vi "Apply Light-Dark Controls Visibility.vi"(8 "Error In":errorcluster, 9 "Dark Controls":refnum<vi>[](array[refnum]), 10 "Light Controls":refnum<vi>[](array[refnum]), 11 "ini Theme in":refnum<class "ini Theme.lvclass">) -> (0 "Error Out":errorcluster, 3 "ini Theme out":refnum<class "ini Theme.lvclass">)   [LabVIEW 2021, in "Appearance Actor.lvlib" / "ini Theme.lvclass"]
doc: "If the loaded theme Type is \"Light\", set <B>Light Controls</B> visibility property to True and <B>Dark Controls</B> ones to False. Else, if \"Dark\", do the other way around."
uses:
  ini Theme.lvclass
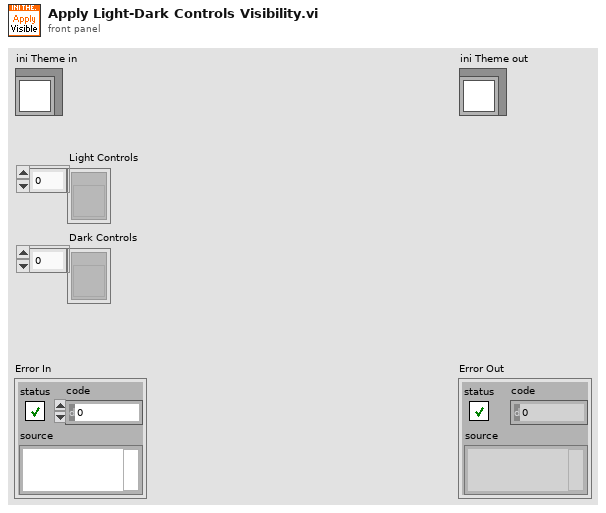
[diagram p1: front panel]
types:
  T1 = typedef "Appearance Actor.lvlib/Generic Theme.lvclass/Theme Info--cluster.ctl" = cluster{"Name":string, "Type":string, "Version":string}
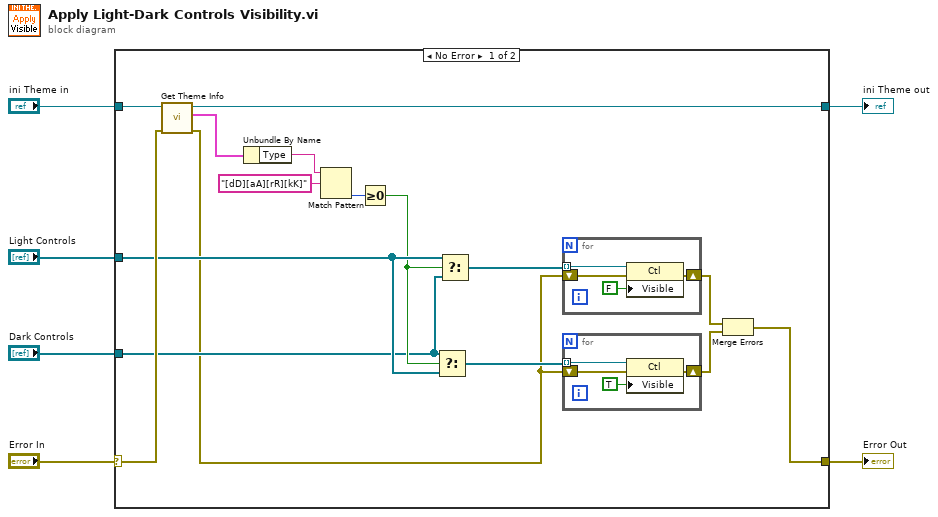
[diagram p0: block diagram]
diagram:
  n1 = case shown="No Error" "Error In" {
    selector: "Error In" -> [w19 w32]
    tunnel: "ini Theme in" -> [w22 w31]
    tunnel: [w21 w31] -> w5
    tunnel: "Light Controls" -> [w15 _]
    tunnel: "Dark Controls" -> [w13 _]
    tunnel: [w7 w32] -> w1
    frame No Error {
      n2 = call-dynamic "Get Theme Info.vi"("Error In"=w19, "ini Theme in"=w22) -> ("Error Out"=w10:errorcluster, "Theme Info"=w20:T1, "ini Theme out"=w21:refnum<class "ini Theme.lvclass">)  [unwired: 7 in]
      n3 = Unbundle By Name(w20) -> ("Type"=w18:string)
      n4 = Match Pattern(string=w18, regular expression="[dD][aA][rR][kK]") -> (offset past match=w16:i32)  [unwired: 1 in, 3 out]
      n5 = Greater Or Equal To 0?(x=w16) -> (x >= 0?=w14:bool)
      n6 = Select(t=w13, s=w14, f=w15) -> (s? t:f=w11:refnum<vi>[])
      n7 = Select(t=w15, s=w14, f=w13) -> (s? t:f=w12:refnum<vi>[])
      n8 = for {
        tunnel: w12 -> [w30] mode=indexing
        shift-right: [w28] -> w9
        shift-left: w10 -> [w27]
        n9 = property class="Ctl"(reference=w30, error in=w27, "Visible"=FALSE) -> (error out=w28:errorcluster)  [unwired: 1 out]
      }
      n10 = for {
        tunnel: w11 -> [w26] mode=indexing
        shift-right: [w24] -> w8
        shift-left: w10 -> [w23]
        n11 = property class="Ctl"(reference=w26, error in=w23, "Visible"=TRUE) -> (error out=w24:errorcluster)  [unwired: 1 out]
      }
      n12 = Merge Errors(w9, w8) -> (w7:errorcluster)
    }
    frame Error {
    }
  }
  "Error Out" <- w1
  "ini Theme out" <- w5
